vi "launcher.vi"() -> ()   [LabVIEW 2021]
panel:
  out "Progress":u8(slide) scale=0.0..100.0
  out "status:":string
  # "Launcher for Distillation Experiment"
  # "100%"
  # "0"
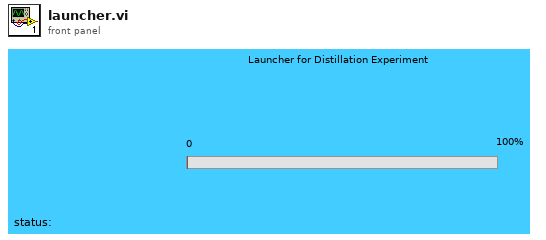
[diagram p1: front panel]
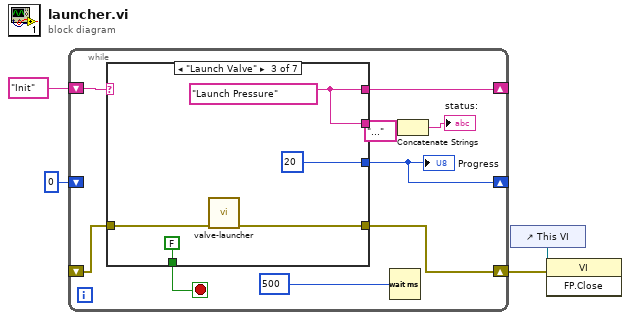
[diagram p0: block diagram]
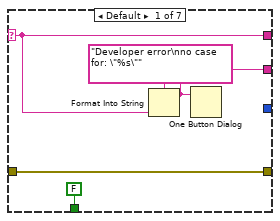
[diagram p2: hidden frame]
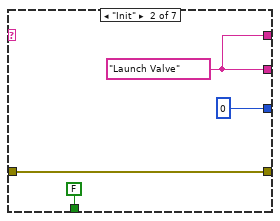
[diagram p3: hidden frame]
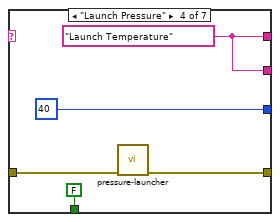
[diagram p4: hidden frame]
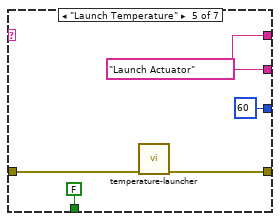
[diagram p5: hidden frame]
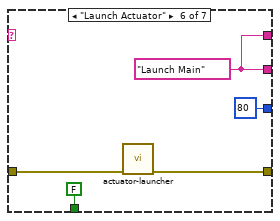
[diagram p6: hidden frame]
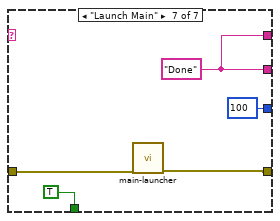
[diagram p7: hidden frame]
diagram:
  n1 = while {
    shift-right: [w11] -> _
    shift-left: u8 0 ("Progress") -> [_]
    shift-right: [w12] -> w3
    shift-left: _ -> [w9]
    shift-right: [w10] -> _
    shift-left: "Init" -> [w13]
    stop <- w5 stop-if-true
    n2 = case shown="\"Launch Valve\"" w13 {
      selector: w13 -> [w17 _ _ _ _ _ _]
      tunnel: [w19 w23 w25 w30 w36 w41 w47] -> w12
      tunnel: [_ u8 0 ("Progress") u8 20 ("Progress") u8 40 ("Progress") u8 60 ("Progress") u8 80 ("Progress") u8 100 ("Progress")] -> w11
      tunnel: [w17 w21 w27 w32 w38 w43 w46] -> w10
      tunnel: w9 -> [w19 w23 w26 w31 w37 w42 w48]
      tunnel: [w16 w21 w27 w32 w38 w43 w46] -> w8
      tunnel: [FALSE FALSE FALSE FALSE FALSE FALSE TRUE] -> w5
      frame Default {
        n3 = Format Into String(format string="Developer error\nno case for: \"%s\"" ("message"), w17) -> (resulting string=w16:string)  [unwired: 2 in, 1 out]
        n4 = One Button Dialog(message=w16) -> ()  [unwired: 1 in, 1 out]
      }
      frame "Init" {
        w21 = "Launch Valve"
      }
      frame "Launch Valve" {
        w27 = "Launch Pressure"
        n5 = call "valve-launcher.vi"("error in (no error)"=w26) -> ("error out"=w25:errorcluster)  [unwired: 10 in]
      }
      frame "Launch Pressure" {
        w32 = "Launch Temperature"
        n6 = call "pressure-launcher.vi"("error in (no error)"=w31) -> ("error out"=w30:errorcluster)  [unwired: 10 in]
      }
      frame "Launch Temperature" {
        w38 = "Launch Actuator"
        n7 = call "temperature-launcher.vi"("error in (no error)"=w37) -> ("error out"=w36:errorcluster)  [unwired: 10 in]
      }
      frame "Launch Actuator" {
        w43 = "Launch Main"
        n8 = call "actuator-launcher.vi"("error in (no error)"=w42) -> ("error out"=w41:errorcluster)  [unwired: 10 in]
      }
      frame "Launch Main" {
        w46 = "Done"
        n9 = call "main-launcher.vi"("error in (no error)"=w48) -> ("error out"=w47:errorcluster)  [unwired: 10 in]
      }
    }
    "Progress" <- w11
    n10 = Wait (ms)(milliseconds to wait=u32 500) -> ()  [unwired: 1 out]
    n11 = Concatenate Strings(w8, "..." ("string")) -> (→"status:":string)
  }
  n12 = control-ref of="This VI"() -> (w4:refnum<vi>)
  n13 = invoke class="VI" method="FP.Close"(reference=w4, error in=w3) -> ()  [unwired: 1 in, 3 out]
